vi "ZL300 Stage Engine.vi"(0 "Notifier Name":string="Not a Name", 11 "Unused Array":string[](array[string])) -> ()   [LabVIEW 2020]
uses:
  Stages Controls/Stage Focus Control.ctl
  Stages Controls/Stage Status.ctl
  Stages Controls/Stage Notifier Element.ctl
  Stages Controls/Stage Actions.ctl
  802b6b2e-b206-4eef-876c-20acfde222b8.vi
  766e80bd-cd52-4e96-a2cb-e966042ef72f.vi
  MCL Libraries/Madlib.dll
panel:
  in  "Direct Move":dbl
  out "Steps":i32
  in  "Get Position":bool
  out "Status":T1
  in  "QUIT":bool
  in  "Focus Control":T2
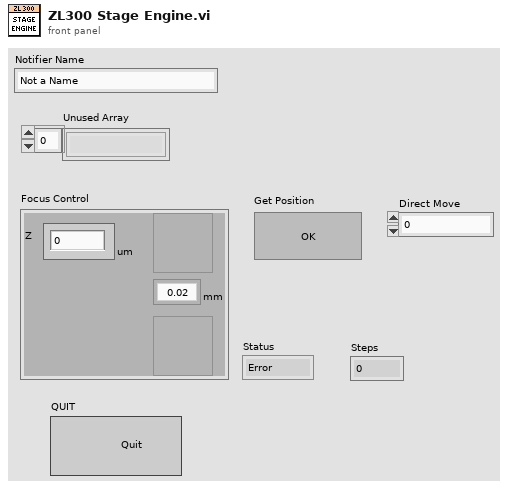
[diagram p1: front panel]
types:
  T1 = typedef "Stage Status.ctl" = enum16{"Error", "Abort", "Busy", "On Target"}
  T2 = typedef "Stage Focus Control.ctl" = cluster{"Focus Step (um)":enum16{"0.02", "0.05", "0.1", "0.5", "1", "2", "5", "10", "20"}, "Focus Up":bool, "Focus Down":bool, "Z ":dbl}
  T3 = typedef "Stage Notifier Element.ctl" = cluster{"Action":T4, "Axis":bool[], "Setpoint":dbl[], "Velocity":dbl, "Cmd Recvd?":bool, "Position":dbl[], "Status":T1, "Misc":variant}
  T4 = typedef "Stage Actions.ctl" = enum16{"Get Position", "MVR", "MOVE", "HALT", "ONTARGET", "ERROR", "REFERENCE", "INIT", "VELOCITY", "STATUS", "EXIT", "HOME", "ZEROPOS", "NANOPOS", "ANALOG", "QUIT"}
  T5 = enum32{"Invalid", "Standard", "Closed", "Hidden", "Minimized", "Maximized"}
  T6 = cluster{"Focus Step (um)":bool, "Focus Up":bool, "Focus Down":bool, "Z ":bool}
  T7 = enum16{"0.02", "0.05", "0.1", "0.5", "1", "2", "5", "10", "20"}
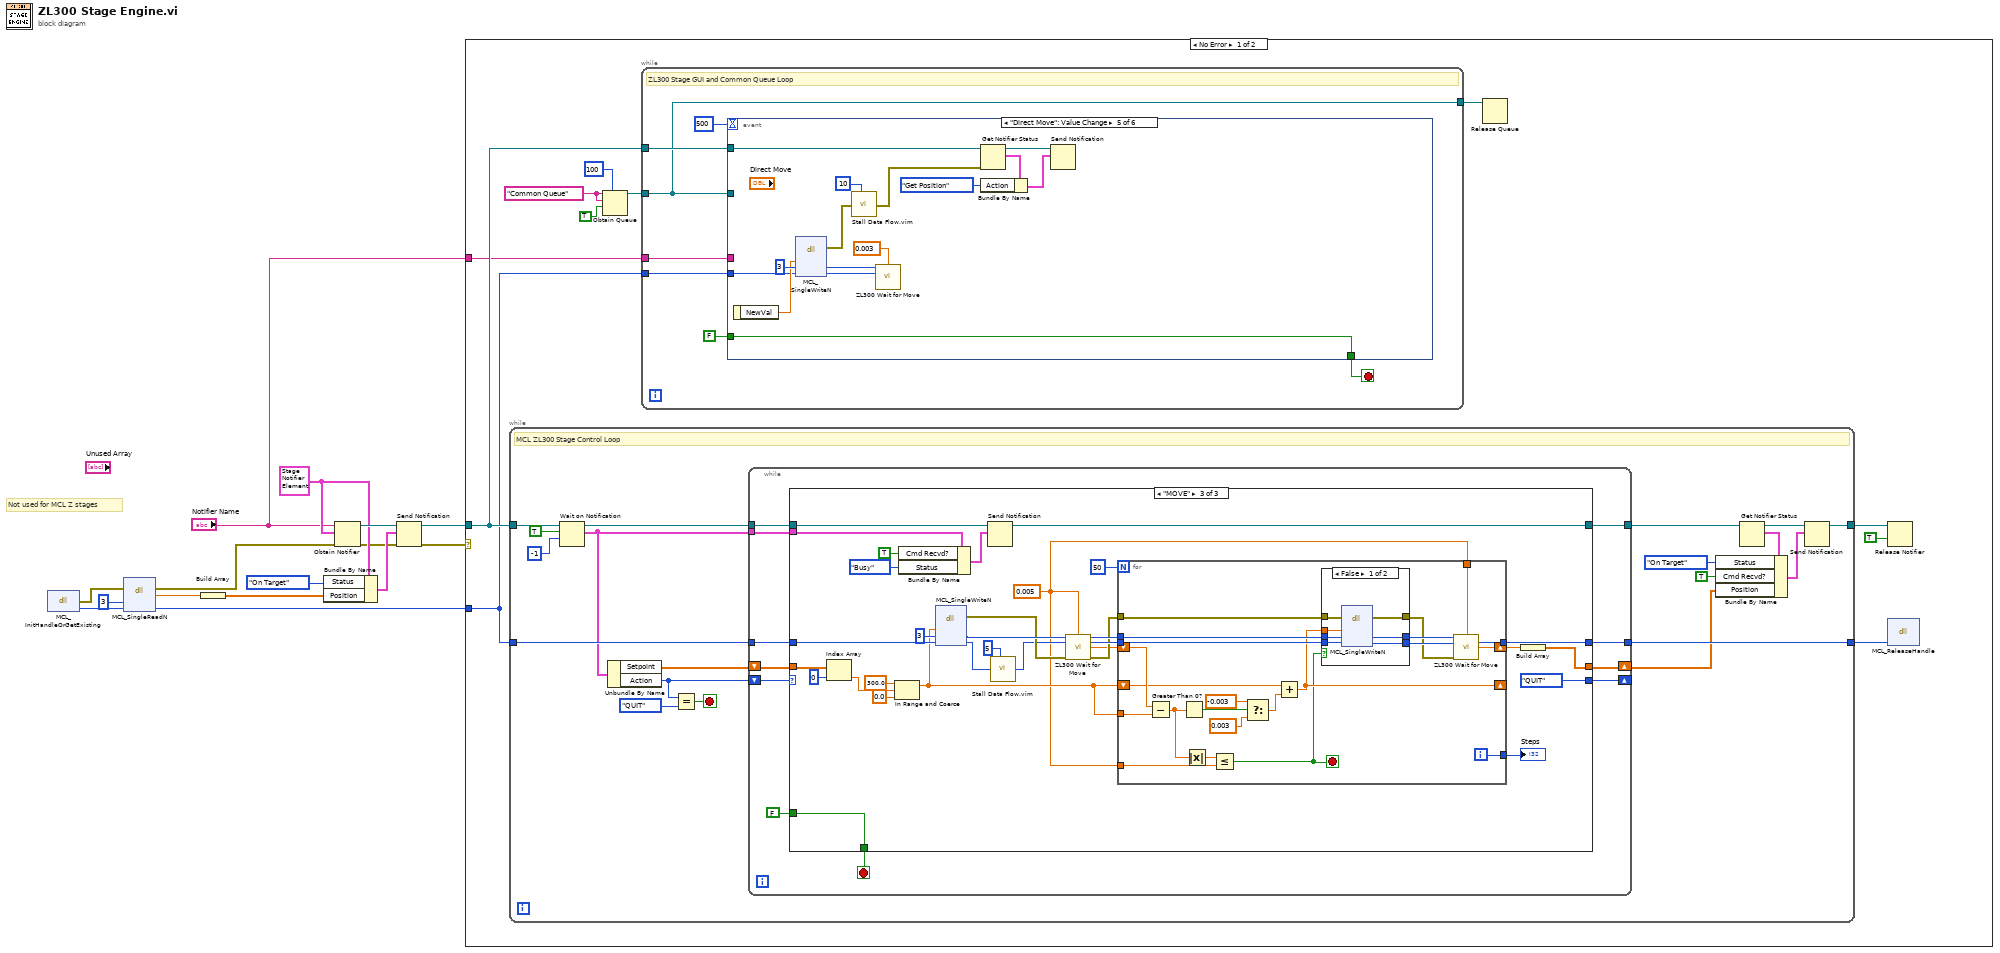
[diagram p0: block diagram]
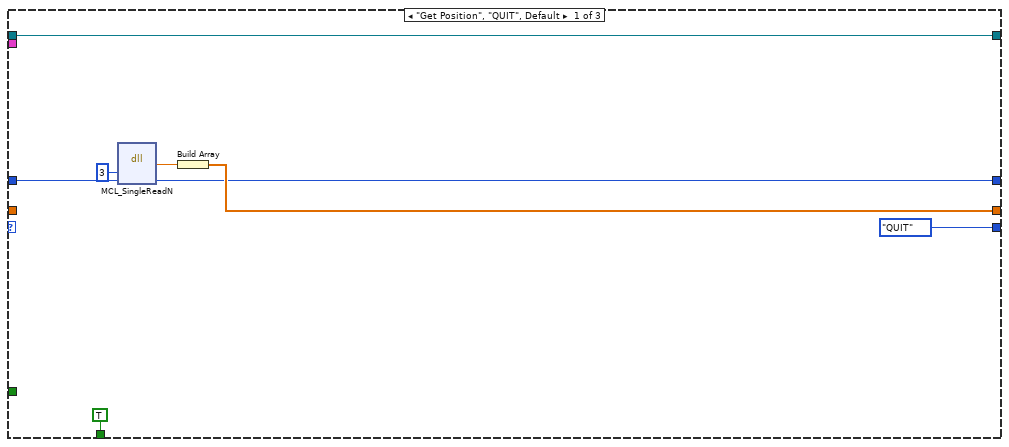
[diagram p2: hidden frame]
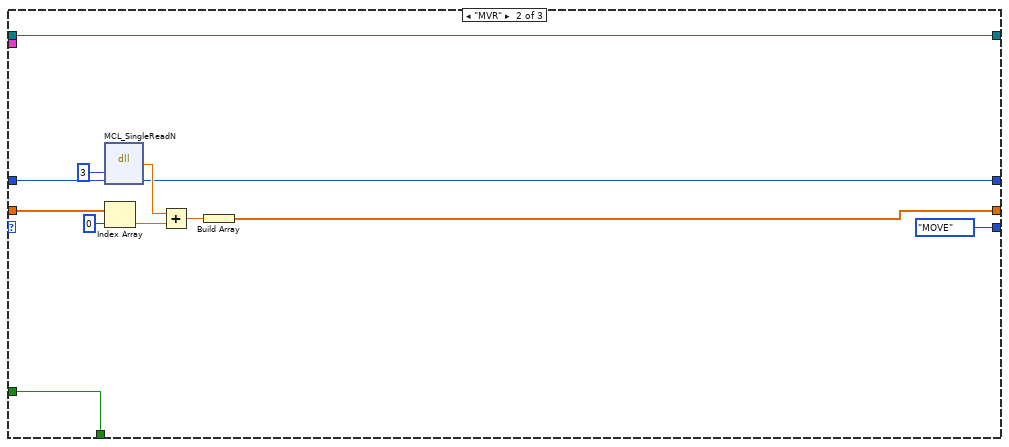
[diagram p3: hidden frame]
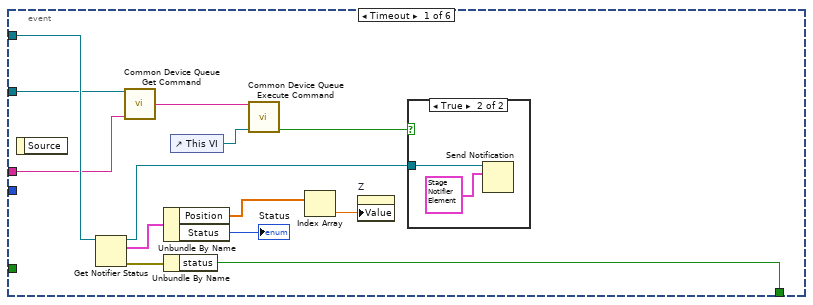
[diagram p5: hidden frame]
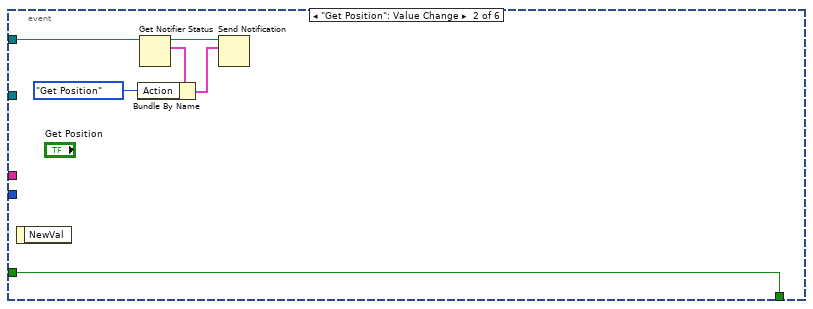
[diagram p7: hidden frame]
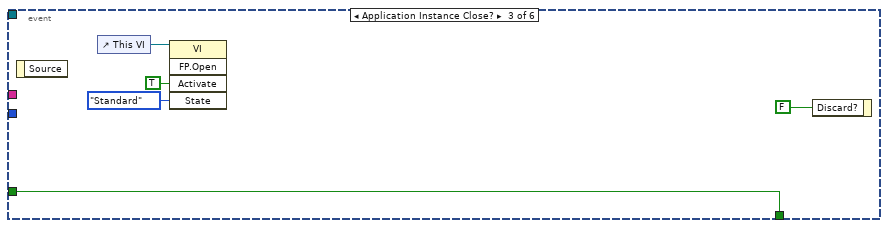
[diagram p8: hidden frame]
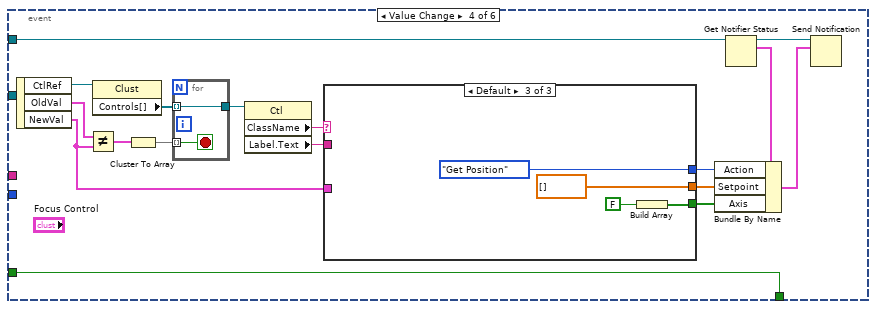
[diagram p9: hidden frame]
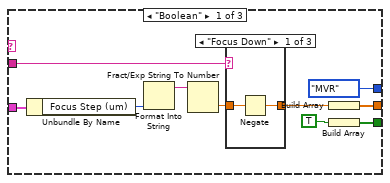
[diagram p10: hidden frame]
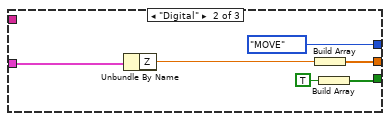
[diagram p13: hidden frame]
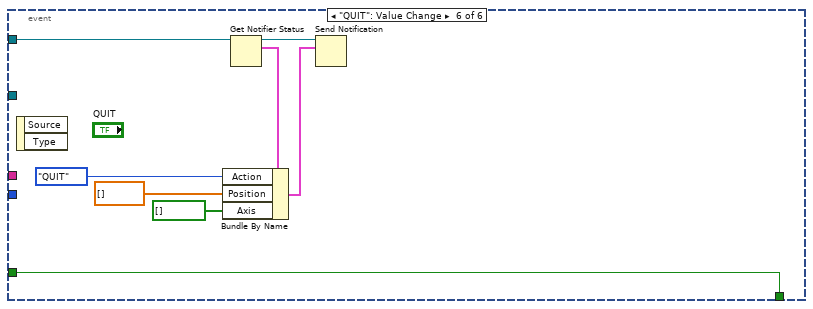
[diagram p14: hidden frame]
diagram:
  w11 = T3 {"Action"=enum."Get Position", "Axis"=[], "Setpoint"=[], "Velocity"=0.5, "Cmd Recvd?"=FALSE, "Position"=[], "Status"=enum."Abort", "Misc"=variant} ("Stage Status")
  # "Not used for MCL Z stages"
  n1 = dll-call lib="C:/Users/George Sirinakis/Documents/Microscope-Control/Device Library/Stages/Mad City Labs/ZL300/MCL Libraries/MADLib.dll" fn="MCL_InitHandleOrGetExisting"() -> (error out=w5:errorcluster, w6:i32)  [unwired: 3 in, 1 out]
  n2 = dll-call lib="C:/Users/George Sirinakis/Documents/Microscope-Control/Device Library/Stages/Mad City Labs/ZL300/MCL Libraries/MADLib.dll" fn="MCL_SingleReadN"(error in=w5, "axis"=u32 3, "handle"=w6) -> (error out=w4:errorcluster, "return type"=w13:dbl, "handle"=w15:i32)  [unwired: 3 in, 1 out]
  n3 = Build Array(w13) -> (w8:dbl[])
  n4 = Bundle By Name(cluster=w11, "Status"=Stage_Status."On Target", "Position"=w8) -> (w10:T3)
  n5 = Obtain Notifier(name (unnamed)="Notifier Name", notification data type=w11, error in (no error)=w4) -> (notifier out=w12:refnum<notifier>, error out=w3:errorcluster)  [unwired: 1 in, 1 out]
  n6 = Send Notification(notification=w10, notifier=w12, error in (no error)=w3) -> (notifier out=w9:refnum<notifier>, error out=w2:errorcluster)
  n7 = case shown="No Error" w2 {
    tunnel: w15 -> [w16 _]
    tunnel: w9 -> [w25 _]
    tunnel: "Notifier Name" -> [w18 _]
    frame No Error {
      w22 = "Common Queue" ("Unique Notifier Name")
      n8 = while {
        tunnel: w16 -> [w39]
        tunnel: [w28] -> w23
        tunnel: w25 -> [w43]
        tunnel: [w34] -> w24
        stop <- w45 stop-if-true
        # "MCL ZL300 Stage Control Loop"
        n9 = Wait on Notification(notifier=w43, ignore previous (F)=TRUE, timeout in ms (-1)=-1) -> (notifier out=w33:refnum<notifier>, notification=w32:T3)  [unwired: 1 in, 2 out]
        n10 = Unbundle By Name(w32) -> ("Setpoint"=w35:dbl[], "Action"=w40:T4)
        n11 = Equal?(x=w40, y=Stage_Actions."QUIT") -> (x = y?=w45:bool)
        n12 = while {
          tunnel: w39 -> [w55]
          tunnel: [w53] -> w28
          shift-right: [w50] -> _
          shift-left: w40 -> [w56]
          tunnel: w33 -> [w49]
          tunnel: w32 -> [w48]
          tunnel: [w47] -> w31
          shift-right: [w46] -> w27
          shift-left: w35 -> [w54]
          stop <- w51 stop-if-true
          n13 = case shown="\"MOVE\"" w56 {
            tunnel: w55 -> [w64 w76 w107]
            tunnel: [w61 w66 w103] -> w46
            tunnel: w54 -> [_ w74 w104]
            tunnel: [w60 w67 w106] -> w53
            tunnel: FALSE -> [_ w72 w102]
            tunnel: [TRUE w72 w102] -> w51
            tunnel: [Stage_Actions."QUIT" ("y") Stage_Actions."MOVE" ("y") Stage_Actions."QUIT" ("y")] -> w50
            tunnel: w49 -> [w58 w65 w87]
            tunnel: w48 -> [_ _ w85]
            tunnel: [w58 w65 w86] -> w47
            frame "Get Position", "QUIT", Default {
              n14 = dll-call lib="C:/Users/George Sirinakis/Documents/Microscope-Control/Device Library/Stages/Mad City Labs/ZL300/MCL Libraries/MADLib.dll" fn="MCL_SingleReadN" label="SingleReadN"("Axis"=u32 3 ("axis"), "Handle"=w64) -> ("Position"=w62:dbl, "Handle"=w60:i32)  [unwired: 4 in, 2 out]
              n15 = Build Array(w62) -> (w61:dbl[])
            }
            frame "MVR" {
              n16 = dll-call lib="C:/Users/George Sirinakis/Documents/Microscope-Control/Device Library/Stages/Mad City Labs/ZL300/MCL Libraries/MADLib.dll" fn="MCL_SingleReadN" label="SingleReadN"("Axis"=u32 3 ("axis"), "Handle"=w76) -> ("Position"=w69:dbl, "Handle"=w67:i32)  [unwired: 4 in, 2 out]
              n17 = Index Array(array=w74, index=0) -> (element=w70:dbl)
              n18 = Add(x=w69, y=w70) -> (x+y=w68:dbl)
              n19 = Build Array(w68) -> (w66:dbl[])
            }
            frame "MOVE" {
              w77 = 0.005 ("Threshold")
              n20 = Index Array(array=w104, index=0) -> (element=w81:dbl)
              n21 = In Range and Coerce(upper limit=300.0, x=w81, lower limit=0.0) -> (coerced(x)=w80:dbl)  [unwired: 1 out]
              n22 = Bundle By Name(cluster=w85, "Cmd Recvd?"=TRUE, "Status"=Stage_Status."Busy") -> (w84:T3)
              n23 = dll-call lib="C:/Users/George Sirinakis/Documents/Microscope-Control/Device Library/Stages/Mad City Labs/ZL300/MCL Libraries/MADLib.dll" fn="MCL_SingleWriteN" label="SingleWriteN"("Position"=w80, "Axis"=u32 3 ("axis"), "Handle"=w107) -> (error out=w97:errorcluster, "Axis"=w98:u32, "Handle"=w99:i32)  [unwired: 5 in, 1 out]
              n24 = Send Notification(notification=w84, notifier=w87) -> (notifier out=w86:refnum<notifier>)  [unwired: 1 in, 1 out]
              n25 = call "Stall Data Flow.vim"("value in"=w99, "milliseconds to wait"=u32 5) -> ("value out"=w90:i32)  [unwired: 1 out]
              n26 = call "ZL300 Wait for Move.vi"("Axis In"=w98, "Threshold"=w77, "Handle In"=w90, "Error In"=w97) -> ("Axis Out"=w96:u32, "Handle Out"=w95:i32, "Position"=w92:dbl, "Error Out"=w94:errorcluster)  [unwired: 8 in]
              n27 = for {
                N: 50 -> [_]
                tunnel: w96 -> [w129]
                tunnel: w94 -> [w124]
                tunnel: w95 -> [w128]
                tunnel: [w125] -> w106
                shift-right: [w116] -> w88
                shift-left: w92 -> [w120]
                shift-right: [w115] -> _
                shift-left: w80 -> [w113]
                tunnel: w80 -> [w112]
                tunnel: [w110] -> w89
                tunnel: w77 -> [w109]
                tunnel: w77 -> [w108]
                i -> [w110]
                stop <- w114 stop-if-true
                n28 = Subtract(x=w120, y=w112) -> (x-y=w118:dbl)
                n29 = Greater Than 0?(x=w118) -> (x > 0?=w123:bool)
                n30 = Absolute Value(x=w118) -> (abs(x)=w117:dbl)
                n31 = Less Or Equal?(x=w117, y=w109) -> (x <= y?=w114:bool)
                n32 = Select(t=-0.003, s=w123, f=0.003) -> (s? t:f=w119:dbl)
                n33 = Add(x=w113, y=w119) -> (x+y=w115:dbl)
                n34 = case shown="False" w114 {
                  tunnel: w129 -> [w136 w138]
                  tunnel: w128 -> [w135 w137]
                  tunnel: [w134 w138] -> w127
                  tunnel: [w133 w137] -> w126
                  tunnel: [w132 w139] -> w111
                  tunnel: w124 -> [w131 w139]
                  tunnel: w115 -> [w130 _]
                  frame False {
                    n35 = dll-call lib="C:/Users/George Sirinakis/Documents/Microscope-Control/Device Library/Stages/Mad City Labs/ZL300/MCL Libraries/MADLib.dll" fn="MCL_SingleWriteN" label="SingleWriteN"(error in=w131, "Position"=w130, "Axis"=w136, "Handle"=w135) -> (error out=w132:errorcluster, "Axis"=w134:u32, "Handle"=w133:i32)  [unwired: 4 in, 1 out]
                  }
                  frame True {
                  }
                }
                n36 = call "ZL300 Wait for Move.vi"("Axis In"=w127, "Threshold"=w108, "Handle In"=w126, "Error In"=w111) -> ("Handle Out"=w125:i32, "Position"=w116:dbl)  [unwired: 8 in, 2 out]
              }
              "Steps" <- w89
              n37 = Build Array(w88) -> (w103:dbl[])
            }
          }
        }
        n38 = Get Notifier Status(notifier=w31) -> (notifier out=w29:refnum<notifier>, current notification=w30:T3)  [unwired: 1 in, 3 out]
        n39 = Bundle By Name(cluster=w30, "Status"=Stage_Status."On Target", "Cmd Recvd?"=TRUE, "Position"=w27) -> (w38:T3)
        n40 = Send Notification(notification=w38, notifier=w29) -> (notifier out=w34:refnum<notifier>)  [unwired: 1 in, 1 out]
      }
      n41 = Obtain Queue(max queue size (-1, unlimited)=100, name (unnamed)=w22, element data type=w22, create if not found? (T)=TRUE) -> (queue out=w19:refnum<queue>)  [unwired: 1 in, 2 out]
      n42 = while {
        tunnel: w25 -> [w144]
        tunnel: w19 -> [w141]
        tunnel: w18 -> [w142]
        tunnel: [w141] -> w17
        tunnel: w16 -> [w140]
        stop <- w145 stop-if-true
        # "ZL300 Stage GUI and Common Queue Loop"
        n43 = event shown="[4] \"Direct Move\": Value Change" {
          selector: _ -> [_ _ _ _ _ _]
          dyn-events: _ -> [_ _ _ _ _ _]
          timeout: 500 -> [_ _ _ _ _ _]
          tunnel: [w159 w167 w168 w173 w230 w231] -> w145
          tunnel: w144 -> [w157 w165 _ w178 w220 w235]
          tunnel: FALSE ("status") -> [_ w167 w168 w173 w230 w231]
          tunnel: w141 -> [w149 _ _ _ _ _]
          tunnel: w142 -> [w147 _ _ _ _ _]
          tunnel: w140 -> [_ _ _ _ w227 _]
          event Timeout {
            n44 = event-data() -> ()  [unwired: 1 in, 1 out]
            n45 = Get Notifier Status(notifier=w157) -> (notifier out=w148:refnum<notifier>, current notification=w156:T3, error out=w154:errorcluster)  [unwired: 1 in, 2 out]
            n46 = call "Common Device Queue Get Command.vi"("Common Queue"=w149, "Notifier Name"=w147) -> ("Command"=w150:string)  [unwired: 12 in, 1 out]
            n47 = Unbundle By Name(w156) -> ("Position"=w155:dbl[], "Status"=→"Status":T1)
            n48 = Unbundle By Name(w154) -> ("status"=w159:bool)
            n49 = control-ref of="This VI"() -> (w151:refnum<vi>)
            n50 = call "Common Device Queue Execute Command.vi"("Common Command"=w150, "VI Refnum"=w151) -> ("Quit?"=w152:bool)  [unwired: 12 in, 1 out]
            n51 = Index Array(array=w155) -> (element=w158:dbl)  [unwired: 1 in]
            n52 = property on="Z" class="DigNum (strict)"("Value"=w158) -> ()  [unwired: 2 in, 2 out]
            n53 = case shown="True" w152 {
              tunnel: w148 -> [_ w161]
              frame False {
              }
              frame True {
                n54 = Send Notification(notification=T3 {"Action"=enum."QUIT", "Axis"=[], "Setpoint"=[], "Velocity"=0.5, "Cmd Recvd?"=FALSE, "Position"=[], "Status"=enum."Error", "Misc"=variant} ("Stage Status"), notifier=w161) -> ()  [unwired: 1 in, 2 out]
              }
            }
          }
          event "Get Position": Value Change {
            n55 = event-data() -> ()  [unwired: 1 in, 1 out]
            n56 = Get Notifier Status(notifier=w165) -> (notifier out=w166:refnum<notifier>, current notification=w164:T3)  [unwired: 1 in, 3 out]
            n57 = Bundle By Name(cluster=w164, "Action"=Stage_Actions."Get Position") -> (w162:T3)
            n58 = Send Notification(notification=w162, notifier=w166) -> ()  [unwired: 1 in, 2 out]
          }
          event Application Instance Close? {
            n59 = event-data() -> ()  [unwired: 1 in, 1 out]
            n60 = control-ref of="This VI"() -> (w170:refnum<vi>)
            n61 = invoke class="VI" method="FP.Open"(reference=w170, "Activate"=TRUE ("Activate?"), "State"=T5."Standard") -> ()  [unwired: 2 in, 5 out]
            n62 = event-data("Discard?"=FALSE) -> ()  [unwired: 1 in, 1 out]
          }
          event Value Change {
            n63 = event-data() -> ("CtlRef"=w188:refnum<vi>, "OldVal"=w189:T2, "NewVal"=w182:T2)  [unwired: 1 in]
            n64 = Not Equal?(x=w189, y=w182) -> (x != y?=w187:T6)
            n65 = property class="Clust"(reference=w188) -> ("Controls[]"=w185:refnum<vi>[])  [unwired: 1 in, 2 out]
            n66 = Cluster To Array(cluster=w187) -> (array=w186:bool[])
            n67 = for {
              tunnel: w186 -> [w215] mode=indexing
              tunnel: [w214] -> w184
              tunnel: w185 -> [w214] mode=indexing
              stop <- w215 stop-if-true
            }
            n68 = property class="Ctl"(reference=w184) -> ("ClassName"=w183:string, "Label.Text"=w181:string)  [unwired: 1 in, 2 out]
            n69 = case shown="Default" w183 {
              tunnel: w182 -> [w197 w209 _]
              tunnel: w181 -> [w198 _ _]
              tunnel: [w192 w207 dbl[] []] -> w180
              tunnel: [w191 w206 w212] -> w179
              tunnel: [Stage_Actions."MVR" ("Action") Stage_Actions."MOVE" ("Action") Stage_Actions."Get Position" ("Action")] -> w177
              frame "Boolean" {
                n70 = Unbundle By Name(w197) -> ("Focus Step (um)"=w195:T7)
                n71 = Format Into String(w195) -> (resulting string=w196:string)  [unwired: 3 in, 1 out]
                n72 = Fract/Exp String To Number(string=w196) -> (number=w194:dbl)  [unwired: 3 in, 1 out]
                n73 = case shown="\"Focus Down\"" w198 {
                  tunnel: w194 -> [w201 w202 w203]
                  tunnel: [w200 w202 w203] -> w193
                  frame "Focus Down" {
                    n74 = Negate(x=w201) -> (-x=w200:dbl)
                  }
                  frame "Focus Up" {
                  }
                  frame Default {
                  }
                }
                n75 = Build Array(w193) -> (w192:dbl[])
                n76 = Build Array(TRUE) -> (w191:bool[])
              }
              frame "Digital" {
                n77 = Unbundle By Name(w209) -> ("Z"=w208:dbl)
                n78 = Build Array(w208) -> (w207:dbl[])
                n79 = Build Array(TRUE) -> (w206:bool[])
              }
              frame Default {
                n80 = Build Array(FALSE) -> (w212:bool[])
              }
            }
            n81 = Get Notifier Status(notifier=w178) -> (notifier out=w176:refnum<notifier>, current notification=w175:T3)  [unwired: 1 in, 3 out]
            n82 = Bundle By Name(cluster=w175, "Action"=w177, "Setpoint"=w180, "Axis"=w179) -> (w174:T3)
            n83 = Send Notification(notification=w174, notifier=w176) -> ()  [unwired: 1 in, 2 out]
          }
          event "Direct Move": Value Change {
            n84 = event-data() -> ("NewVal"=w228:dbl)  [unwired: 1 in]
            n85 = dll-call lib="C:/Users/George Sirinakis/Documents/Microscope-Control/Device Library/Stages/Mad City Labs/ZL300/MCL Libraries/MADLib.dll" fn="MCL_SingleWriteN"("Position"=w228, "Axis"=u32 3 ("axis"), "Handle"=w227) -> (error out=w218:errorcluster, "Axis"=w225:u32, "Handle"=w224:i32)  [unwired: 5 in, 1 out]
            n86 = call "Stall Data Flow.vim"("value in"=w218, "milliseconds to wait"=u32 10) -> ("value out"=w216:errorcluster)  [unwired: 1 out]
            n87 = call "ZL300 Wait for Move.vi"("Axis In"=w225, "Threshold"=0.003, "Handle In"=w224) -> ()  [unwired: 9 in, 4 out]
            n88 = Get Notifier Status(notifier=w220, error in (no error)=w216) -> (notifier out=w223:refnum<notifier>, current notification=w222:T3)  [unwired: 3 out]
            n89 = Bundle By Name(cluster=w222, "Action"=Stage_Actions."Get Position") -> (w221:T3)
            n90 = Send Notification(notification=w221, notifier=w223) -> ()  [unwired: 1 in, 2 out]
          }
          event "QUIT": Value Change {
            n91 = event-data() -> ()  [unwired: 1 in, 2 out]
            n92 = Get Notifier Status(notifier=w235) -> (notifier out=w233:refnum<notifier>, current notification=w232:T3)  [unwired: 1 in, 3 out]
            n93 = Bundle By Name(cluster=w232, "Action"=Stage_Actions."QUIT", "Position"=dbl[] [], "Axis"=bool[] []) -> (w236:T3)
            n94 = Send Notification(notification=w236, notifier=w233) -> ()  [unwired: 1 in, 2 out]
          }
        }
      }
      n95 = Release Queue(queue=w17) -> ()  [unwired: 2 in, 3 out]
      n96 = Release Notifier(notifier=w24, force destroy? (F)=TRUE) -> ()  [unwired: 1 in, 3 out]
      n97 = dll-call lib="C:/Users/George Sirinakis/Documents/Microscope-Control/Device Library/Stages/Mad City Labs/ZL300/MCL Libraries/MADLib.dll" fn="MCL_ReleaseHandle"("handle"=w23) -> ()  [unwired: 5 in, 2 out]
    }
    frame Error {
    }
  }
